vi "Read outputs.vi"(9 "Diagram in":refnum<class "Diagram.lvclass">) -> (3 "Diagram out":refnum<class "Diagram.lvclass">, 4 "outputs":refnum<class "Terminal.lvclass">[](array[class]))   [LabVIEW 2014, in "Diagram.lvclass"]
uses:
  Diagram.lvclass
  Terminal/Terminal.lvclass
  Diagram.lvclass/Diagram.ctl
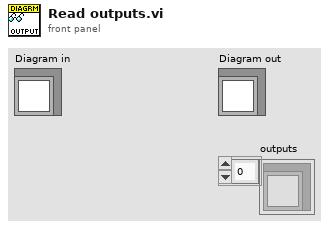
[diagram p1: front panel]
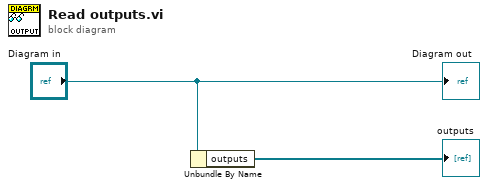
[diagram p0: block diagram]
diagram:
  n1 = Unbundle By Name("Diagram in") -> ("outputs"=→"outputs":refnum<class "Terminal.lvclass">[])
  "Diagram out" <- "Diagram in"
